vi "WPI_Power Get PCM Faults.vi"(0 "Pneumatics Control Module (0)":u8, 5 "Solenoid Channel":T1, 7 "Clear Sticky Faults":bool, 11 "error in":errorcluster) -> (6 "Compressor Fault":bool, 8 "Solenoid Fault":bool, 10 "All Solenoid Faults":bool[](array[boolean]), 15 "error out":errorcluster)   [LabVIEW 2017]
doc: "Returns compressor and solenoid faults on the Pnuematics Control Module (PCM)."
uses:
  <vilib>/Rock Robotics/WPI/Solenoid/WPI_SolenoidChannel.ctl
  <vilib>/Rock Robotics/WPI/CAN/PCM/WPI_CAN_PCMGlobalOps.ctl
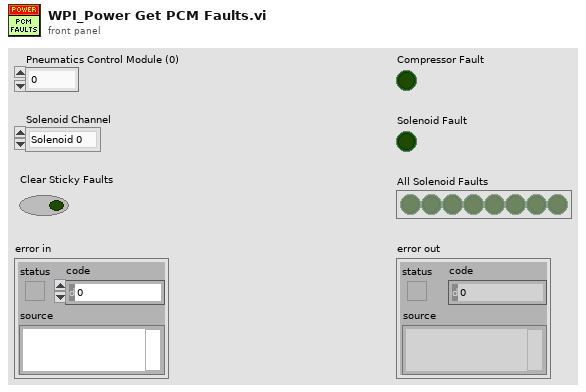
[diagram p1: front panel]
types:
  T1 = typedef "WPI_SolenoidChannel.ctl" = enum8{"Solenoid 0", "Solenoid 1", "Solenoid 2", "Solenoid 3", "Solenoid 4", "Solenoid 5", "Solenoid 6", "Solenoid 7", "Invalid"}
  T2 = typedef "WPI_CAN_PCMGlobalOps.ctl" = enum16{"Read For Send", "Write After Receive", "Set Solenoids", "Set Closed Loop", "Clear Sticky Faults", "Get All", "Write Error", "Write After Receive Blacklist", "Set Control Frame Rate"}
  T3 = cluster{"Solenoid Status":bool[], "Battery Voltage":dbl, "Solenoid Voltage":dbl, "Compressor Current":dbl, "CompressorEnabled":bool, "StickySolenoidFault":bool, "StickyCompressorFault":bool, "SolenoidFault":bool, "CompressorFault":bool, "HardwareFault":bool, "ClosedLoopStatus":bool, "PressureStatus":bool, "Module Enabled":bool, "ClosedLoopSuggestedOutput":bool, "CAN Error":errorcluster, "Sticky Solenoid Faults":bool[]}
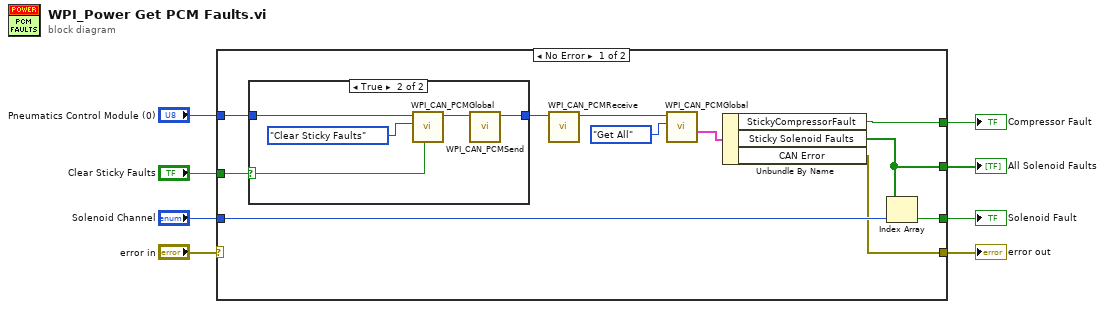
[diagram p0: block diagram]
diagram:
  n1 = case shown="No Error" "error in" {
    selector: "error in" -> [_ w26]
    tunnel: [w9 w26] -> w7
    tunnel: "Pneumatics Control Module (0)" -> [w16 _]
    tunnel: [w13 _] -> w4
    tunnel: "Clear Sticky Faults" -> [w14 _]
    tunnel: "Solenoid Channel" -> [w12 _]
    tunnel: [w11 _] -> w2
    tunnel: [w10 _] -> w1
    frame No Error {
      n2 = case shown="True" w14 {
        selector: w14 -> [_ w24]
        tunnel: w16 -> [w20 w23]
        tunnel: [w20 w21] -> w15
        frame False {
        }
        frame True {
          n3 = call <vilib>:"WPI_CAN_PCMGlobal.vi"("Set Value"=w24, "Operation"=WPI_CAN_PCMGlobalOps."Clear Sticky Faults", "Pneumatics Control Module (0)"=w23) -> ("Pneumatics Control Module Out"=w22:u8)  [unwired: 6 in, 2 out]
          n4 = call <vilib>:"WPI_CAN_PCMSend.vi"("Pneumatics Control Module (0)"=w22) -> ("Pneumatics Control Module Out"=w21:u8)  [unwired: 10 in]
        }
      }
      n5 = call <vilib>:"WPI_CAN_PCMReceive.vi"("Pneumatics Control Module (0)"=w15) -> ("Pneumatics Control Module Out"=w18:u8)  [unwired: 10 in]
      n6 = call <vilib>:"WPI_CAN_PCMGlobal.vi"("Operation"=WPI_CAN_PCMGlobalOps."Get All", "Pneumatics Control Module (0)"=w18) -> ("Get All"=w19:T3)  [unwired: 7 in, 2 out]
      n7 = Unbundle By Name(w19) -> ("StickyCompressorFault"=w10:bool, "Sticky Solenoid Faults"=w13:bool[], "CAN Error"=w9:errorcluster)
      n8 = Index Array(array=w13, index=w12) -> (element=w11:bool)
    }
    frame Error {
    }
  }
  "error out" <- w7
  "All Solenoid Faults" <- w4
  "Solenoid Fault" <- w2
  "Compressor Fault" <- w1
